vi "LWConexPSD_Example.vi"() -> ()   [LabVIEW 2010]
uses:
  C:/Users/LeeGS/Desktop/랩뷰/실험실 노트북/LGS_test/CONEX-PSD9/Dll/Newport.CONEXPSD.CommandInterface.DLL
  Dll/Newport.CONEXPSD.CommandInterface.DLL
panel:
  out "errstring 4":string
  out "outCommandError":string
  out "TB":i32
  out "errstring 3":string
  out "LastCommandError":string
  out "TE":i32
  out "errstring 2":string
  out "controllerState":string
  out "errorCode":string
  out "TS":i32
  out "VE error":i32
  in  "Launch server?":bool=TRUE
  in  "Authorize?":bool=TRUE
  out "Error out":errorcluster caption="error out"
  in  "Instrument Key":string
  out "errstring":string
  out "ControllerVersion":string
  # "컨트롤러 상태 출력"
  # "에러코드 확인"
  # "TS command test"
  # "TE command test"
  # "에러코드를 문자로 변환"
  # "TB command test"
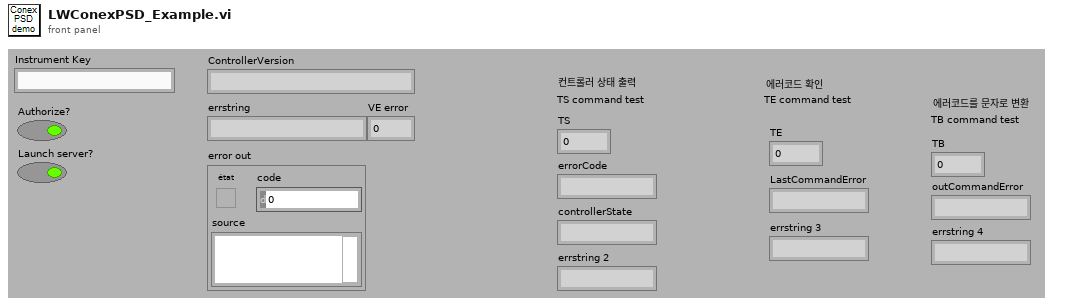
[diagram p1: front panel]
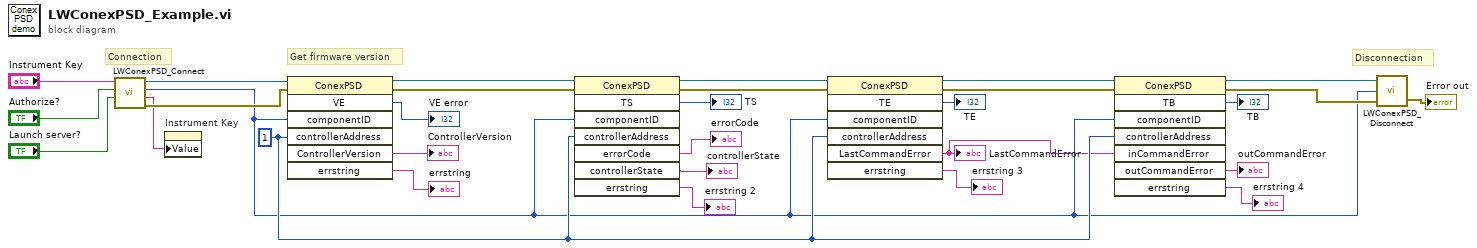
[diagram p0: block diagram]
diagram:
  w6 = 1 ("controllerAddress")
  # "Get firmware version"
  # "Disconnection"
  # "Connection"
  n1 = call "LWConexPSD_Connect.vi"("Launch server? (True)"="Launch server?", "Authorize? (True)"="Authorize?", "Instrument Key"="Instrument Key") -> ("error out"=w29:errorcluster, "Instrument Key out"=w24:string, "Component ID"=w5:i32, "ConexPSD Reference"=w30:refnum<k24>)  [unwired: 1 in]
  n2 = property on="Instrument Key" class="Str"("Value"=w24) -> ()  [unwired: 2 in, 2 out]
  n3 = invoke class="ConexPSD" method="VE"(reference=w30, error in=w29, "componentID"=w5, "controllerAddress"=w6) -> (reference out=w20:refnum<k24>, error out=w19:errorcluster, "VE"=→"VE error":i32, "ControllerVersion"=→"ControllerVersion":string, "errstring"=→"errstring":string)  [unwired: 3 in, 2 out]
  n4 = invoke class="ConexPSD" method="TS"(reference=w20, error in=w19, "componentID"=w5, "controllerAddress"=w6) -> (reference out=w14:refnum<k24>, error out=w13:errorcluster, "TS"=→"TS":i32, "errorCode"=→"errorCode":string, "controllerState"=→"controllerState":string, "errstring"=→"errstring 2":string)  [unwired: 4 in, 2 out]
  n5 = invoke class="ConexPSD" method="TE"(reference=w14, error in=w13, "componentID"=w5, "controllerAddress"=w6) -> (reference out=w10:refnum<k24>, error out=w9:errorcluster, "TE"=→"TE":i32, "LastCommandError"=w2:string, "errstring"=→"errstring 3":string)  [unwired: 3 in, 2 out]
  "LastCommandError" <- w2
  n6 = invoke class="ConexPSD" method="TB"(reference=w10, error in=w9, "componentID"=w5, "controllerAddress"=w6, "inCommandError"=w2) -> (reference out=w8:refnum<k24>, error out=w7:errorcluster, "TB"=→"TB":i32, "outCommandError"=→"outCommandError":string, "errstring"=→"errstring 4":string)  [unwired: 3 in, 3 out]
  n7 = call "LWConexPSD_Disconnect.vi"("error in (no error)"=w7, "Component ID"=w5, "ConexPSD Référence"=w8) -> ("Error out"=→"Error out":errorcluster)  [unwired: 1 in]
